vi "GVHeizenLH_ECD.vi"() -> ()   [LabVIEW 2017]
panel:
  in  "Heizen?LH":bool[](array[boolean])
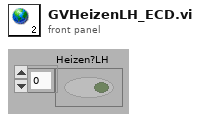
[diagram p1: front panel]
diagram:
